vi "Draw Border.vi"(8 "error in (no error)":errorcluster, 11 "Scalable Border in":refnum<class "Scalable Border.lvclass">) -> (0 "error out":errorcluster, 2 "Border out":picture, 3 "Scalable Border out":refnum<class "Scalable Border.lvclass">)   [LabVIEW 2015, in "Scalable Border.lvclass"]
uses:
  Scalable Border.lvclass
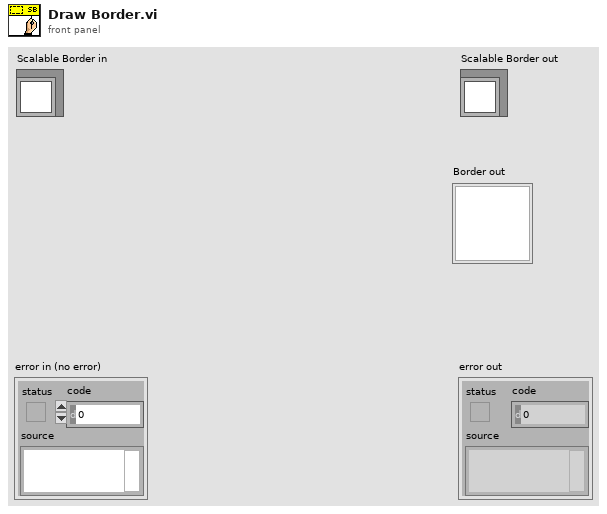
[diagram p1: front panel]
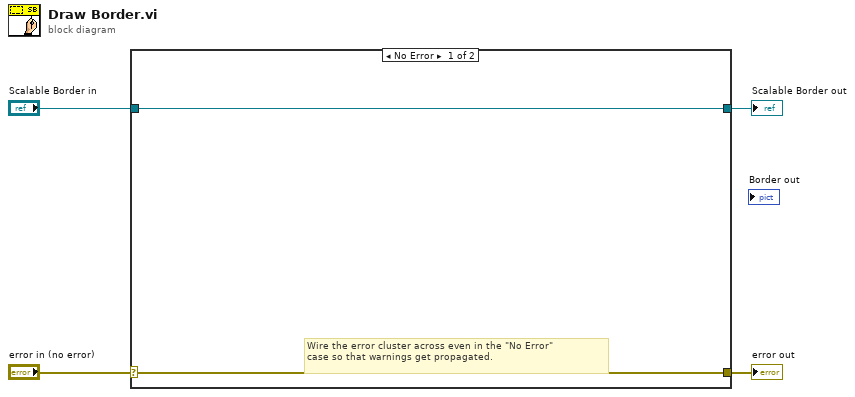
[diagram p0: block diagram]
diagram:
  n1 = case shown="No Error" "error in (no error)" {
    selector: "error in (no error)" -> [w5 w8]
    tunnel: [w5 w8] -> w3
    tunnel: [w6 w7] -> w1
    tunnel: "Scalable Border in" -> [w6 w7]
    frame No Error {
      # "Wire the error cluster across even in the \"No Error\"\ncase so that warnings get propagated."
    }
    frame Error {
    }
  }
  "error out" <- w3
  "Scalable Border out" <- w1
